vi "SV Read Spectra from Data Object.vi"(8 "error in (no error)":errorcluster, 10 "component":T1=32 items=["Magnitude^2"=37, "Magnitude"=32, "Phase"=33, "Real"=34, "Imaginary"=35, "Coherence"=36, "Unknown"=99], 11 "Data in":refnum<class "Data.lvclass">) -> (0 "error out":errorcluster, 1 "spectra info":T2[](array[typedef]) {"x-axis units" items=["Time (s)"=0, "Frequency-CB (Hz)"=1, "Frequency-CPB (Hz)"=1248, "Frequency-Arbitrary (Hz)"=2357, "Quefrency (s)"=2, "Revolutions (rev)"=3, "Order"=4, "Speed (RPM)"=11, "Speed (rad/s)"=21, "Index"=65535]; "weighting filter" items=["Linear", "A-weighting", "B-weighting", "C-weighting", "ITU-R 468-4", "Dolby", "CCITT", "C-message", "Wb", "Wc", "Wd", "We", "Wf", "Wh", "Wj", "Wk", "Wm", "AES17 20 kHz lowpass", "AES17 40 kHz lowpass", "AES17 20 kHz highpass", "AES17 40 kHz highpass"]; "dB reference [EU]" format="%.2f"; "engineering units" items=["custom..."=0, "V"=1, "A"=21, "C"=30, "pC"=31, "s"=32, "-"=29, "Pa"=2, "N"=20, "g"=3, "m/s^2"=4, "m/s"=5, "m"=6, "mm/s"=12, "mm"=13, "micron/s"=14, "micron"=15, "in/s^2"=7, "in/s"=8, "in"=9, "mil/s"=10, "mil"=11, "rad/s^2"=16, "rad/s"=17, "rad"=18, "deg/s^2"=26, "deg/s"=27, "deg"=28, "RPM"=22, "cycle/s^2"=23, "Hz"=24, "cycle"=25, "strain"=19]; "spectral info"."window" items=["None "=0, "Hanning"=1, "Hamming"=2, "Blackman-Harris"=3, "Exact Blackman"=4, "Blackman"=5, "Flat Top"=6, "4 Term B-Harris "=7, "7 Term B-Harris"=8, "Low Sidelobe"=9, "Force - Exponential"=10, "Gaussian"=62]}, 2 "spectra":cluster{"x0":dbl, "dx":dbl, "Y":dbl[]}[](array[cluster]), 3 "Data out":refnum<class "Data.lvclass">, 4 "global attributes":variant)   [LabVIEW 2017]
doc: "This VI always reads N Channel spectra from the data object."
uses:
  <vilib>/addons/_NISVFA/_Shared subVIs/Data Objects/Data/Data.lvclass
  <vilib>/addons/_NISVFA/_Shared subVIs/Controls/svc_Spectrum Info.ctl
  <vilib>/addons/_NISVFA/_Shared subVIs/Controls/svc_X-Axis Units.ctl
  <vilib>/addons/_NISVFA/_Shared subVIs/Controls/svc_Spectrum Type.ctl
  <vilib>/addons/_NISVFA/_Shared subVIs/Controls/svc_Engineering Units Text Ring.ctl
  <vilib>/addons/_NISVFA/_Shared subVIs/Controls/svc_Weighting Filter Text Ring.ctl
  <vilib>/addons/_NISVFA/_Shared subVIs/Controls/svc_Complimentary Spectrum Units.ctl
  <vilib>/addons/_NISVFA/_Shared subVIs/Controls/NI Spectrum Component.ctl
  <vilib>/addons/_NISVFA/_Shared subVIs/Controls/NI Channel Properties.ctl
  <vilib>/addons/_NISVFA/_Shared subVIs/Data Objects/Y (DBL)/Y (1 Ch).lvclass
  C:/Program Files (x86)/National Instruments/LabVIEW 2017/vi.lib/addons/_NISVFA/_Shared subVIs/Data Objects/Data/Data.lvclass
  <vilib>/addons/_NISVFA/_Shared subVIs/Data Objects/Data/Data.lvclass/Data.ctl
  <vilib>/addons/_NISVFA/_Shared subVIs/Data Objects/Y (DBL)/Y (N Ch).lvclass
  <vilib>/addons/_NISVFA/_Shared subVIs/Data Objects/Y (Complex) (DBL)/Y (Complex) (1 Ch).lvclass
  <vilib>/addons/_NISVFA/_Shared subVIs/Data Objects/Y (Complex) (DBL)/Y (Complex) (1 Ch).lvclass/Y (Complex) (1 Ch).ctl
  <vilib>/addons/_NISVFA/_Shared subVIs/Data Objects/Y (Complex) (DBL)/Y (Complex) (N Ch).lvclass
  <vilib>/addons/_NISVFA/_Shared subVIs/Data Objects/Y (Complex) (DBL)/Y (Complex) (N Ch).lvclass/Y (Complex) (N Ch).ctl
  <vilib>/addons/_NISVFA/_Shared subVIs/Common/sv_Get SV Property Name String.vi
  <vilib>/addons/_NISVFA/_Shared subVIs/Common/svc_Spectrum Units.vi
  <vilib>/addons/_NISVFA/_Shared subVIs/Spectrum Info/sfva_Set SV Info in Spectrum Info Description.vi
  <vilib>/addons/_NISVFA/_Shared subVIs/Common/svc_Get Weighting Enum and Labels.vi
  <vilib>/addons/_NISVFA/_Shared subVIs/Common/svc_Unit Label Lexical Class.vi
  <vilib>/addons/_NISVFA/_Shared subVIs/Common/svc_Engineering Units to Unit Label.vi
  <vilib>/addons/_NISVFA/_Shared subVIs/Common/svc_Format Value (DBL).vi
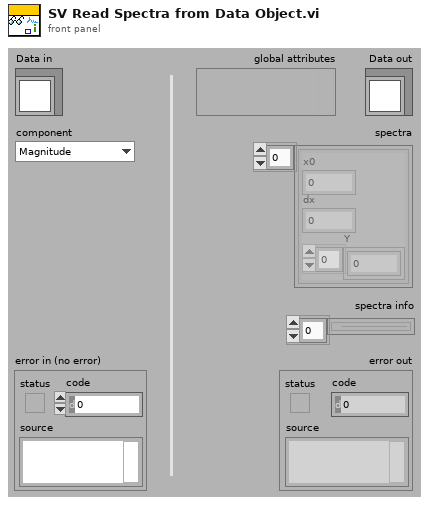
[diagram p1: front panel]
types:
  T1 = typedef "NI Spectrum Component.ctl" = u16
  T2 = typedef "svc_Spectrum Info.ctl" = cluster{"channel name":string, "description":string, "x-axis units":T3, "spectral info":cluster{"spectrum type":T4, "linear/dB":enum16{"linear", "dB"}, "window":u16, "window size":i32, "FFT size":i32}, "engineering units":T5, "custom label":string, "dB reference [EU]":dbl, "peak units":enum16{"rms", "peak", "peak-peak"}, "weighting filter":T6, "spectral density?":bool, "unit label":string, "spectrum skewed?":bool, "complimentary spectrum units":T7}
  T3 = typedef "svc_X-Axis Units.ctl" = u16
  T4 = typedef "svc_Spectrum Type.ctl" = enum16{"FFT Spectrum [complex]", "Amplitude [Magnitude]", "Power [Magnitude^2]", "Cross Spectrum [complex]", "Frequency Response [Complex]"}
  T5 = typedef "svc_Engineering Units Text Ring.ctl" = u16
  T6 = typedef "svc_Weighting Filter Text Ring.ctl" = u16
  T7 = typedef "svc_Complimentary Spectrum Units.ctl" = enum16{"none", "radians", "degrees", "cycles", "imaginary"}
  T8 = typedef "NI Channel Properties.ctl" = u16
  T9 = cluster{"Y":dbl[], "channel attributes":variant}[]
  T10 = cluster{"Y":cdb[], "channel attributes":variant}[]
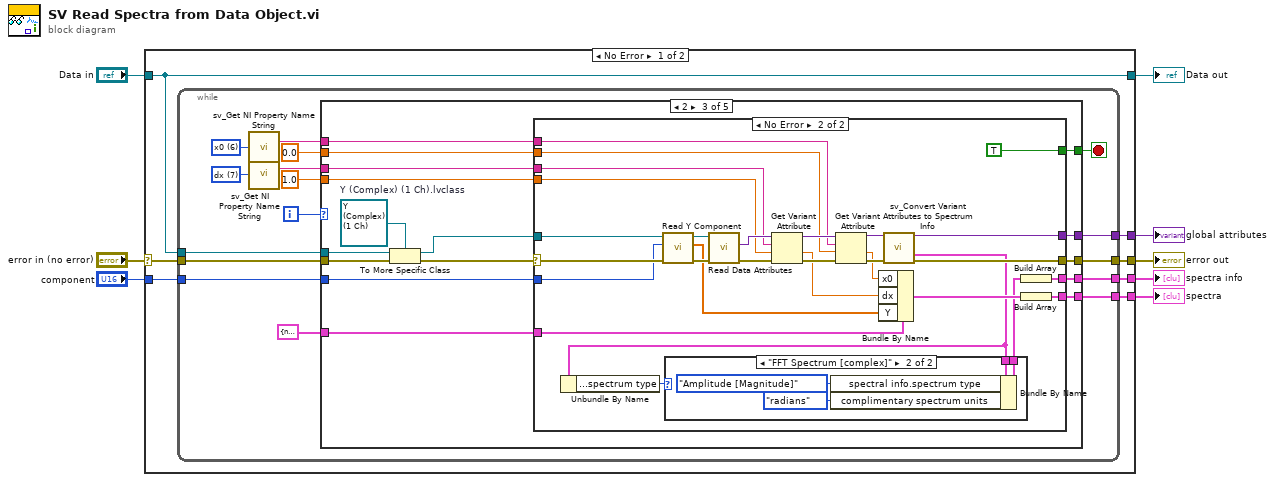
[diagram p0: block diagram]
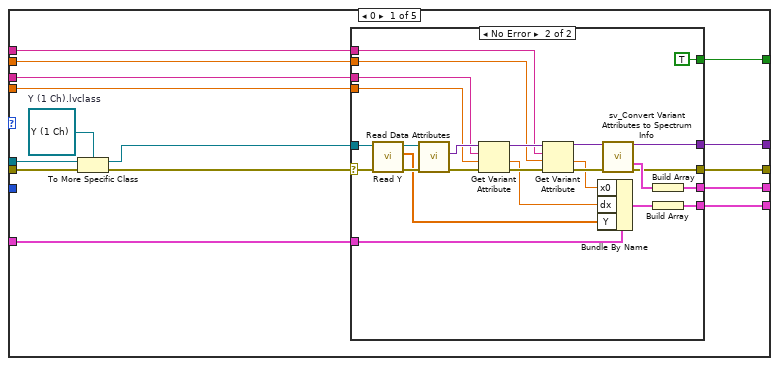
[diagram p2: hidden frame]
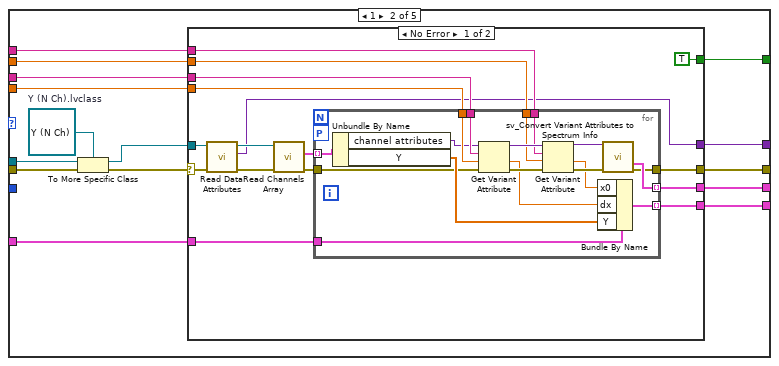
[diagram p4: hidden frame]
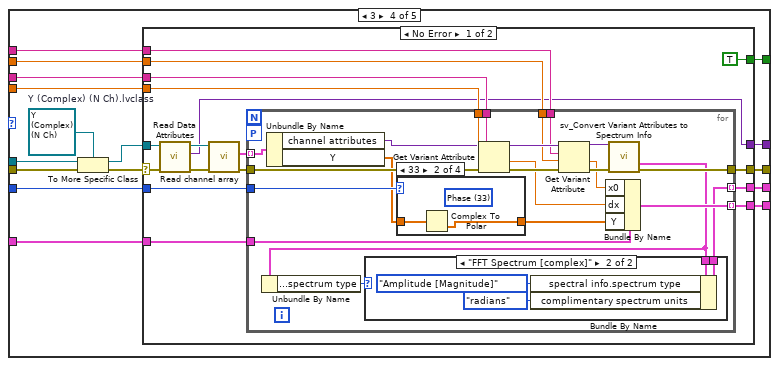
[diagram p8: hidden frame]
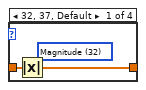
[diagram p10: hidden frame]
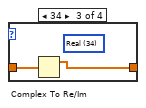
[diagram p11: hidden frame]
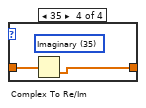
[diagram p12: hidden frame]
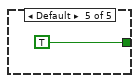
[diagram p14: hidden frame]
diagram:
  n1 = case shown="No Error" "error in (no error)" {
    selector: "error in (no error)" -> [w15 w243]
    tunnel: [w12 w243] -> w7
    tunnel: [w14 w244] -> w5
    tunnel: "Data in" -> [w14 w244]
    tunnel: [w13 _] -> w2
    tunnel: [w11 _] -> w4
    tunnel: [w10 _] -> w3
    tunnel: "component" -> [w9 _]
    frame No Error {
      n2 = while {
        tunnel: [w20] -> w12
        tunnel: w15 -> [w29]
        tunnel: w14 -> [w30]
        tunnel: [w21] -> w13
        tunnel: [w19] -> w11
        tunnel: [w18] -> w10
        tunnel: w9 -> [w16]
        i -> [w31]
        stop <- w17 stop-if-true
        w28 = T8 7 items=["Channel name", "Channel description", "Y-axis label", "Y-axis unit string", "X-axis label", "X-axis unit string", "x0", "dx", "Number of samples", "X channel", "Filter settled", "dB reference", "Window", "Window parameter", "Window size", "FFT size", "Peak units", "Spectrum type", "Magnitude scale", "Spectral density"] ("property")
        w27 = T8 6 items=["Channel name", "Channel description", "Y-axis label", "Y-axis unit string", "X-axis label", "X-axis unit string", "x0", "dx", "Number of samples", "X channel", "Filter settled", "dB reference", "Window", "Window parameter", "Window size", "FFT size", "Peak units", "Spectrum type", "Magnitude scale", "Spectral density"] ("property")
        n3 = call <vilib>:"sv_Get NI Property Name String.vi"("property"=w27) -> ("TDMS property name"=w26:string)  [unwired: 13 in, 1 out]
        n4 = call <vilib>:"sv_Get NI Property Name String.vi"("property"=w28) -> ("TDMS property name"=w24:string)  [unwired: 13 in, 1 out]
        n5 = case shown="2" w31 {
          tunnel: w30 -> [w45 w86 w137 w187 _]
          tunnel: w29 -> [w44 w85 w136 w186 _]
          tunnel: w26 -> [w43 w82 w135 w183 _]
          tunnel: 0.0 -> [w42 w81 w134 w182 _]
          tunnel: w24 -> [w41 w80 w133 w181 _]
          tunnel: 1.0 -> [w40 w79 w132 w180 _]
          tunnel: cluster{"x0":dbl, "dx":dbl, "Y":dbl[]} {"x0"=nan, "dx"=nan, "Y"=[nan]} ("power spectrum [dB EU]") -> [w39 w78 w131 w179 _]
          tunnel: [w36 w74 w128 w175 _] -> w21
          tunnel: [w35 w75 w127 w176 _] -> w20
          tunnel: [w34 w76 w126 w177 _] -> w19
          tunnel: [w33 w77 w125 w178 _] -> w18
          tunnel: [w32 w73 w124 w174 TRUE] -> w17
          tunnel: w16 -> [_ _ w123 w173 _]
          frame 0 {
            w46 = refnum<class "Y (1 Ch).lvclass"> refnum  # Y (1 Ch).lvclass
            n6 = To More Specific Class(target class=w46, reference=w45, error in=w44) -> (specific class reference=w37:refnum<class "Y (1 Ch).lvclass">, error out=w38:errorcluster)
            n7 = case shown="No Error" w38 {
              selector: w38 -> [w47 w52]
              tunnel: w37 -> [_ w61]
              tunnel: [_ w53] -> w34
              tunnel: w43 -> [_ w60]
              tunnel: w41 -> [_ w58]
              tunnel: w40 -> [_ w57]
              tunnel: w42 -> [_ w59]
              tunnel: w39 -> [_ w56]
              tunnel: [_ w55] -> w33
              tunnel: [w47 w51] -> w35
              tunnel: [_ w50] -> w36
              tunnel: [_ TRUE] -> w32
              frame Error {
              }
              frame No Error {
                n8 = call <vilib>:"Read Y.vi"("error in (no error)"=w52, "Y (1Ch) in"=w61) -> ("error out"=w67:errorcluster, "Y"=w62:dbl[], "Y (1Ch) out"=w72:refnum<class "Y (1 Ch).lvclass">)  [unwired: 7 in]
                n9 = call <vilib>:"Read Data Attributes.vi"("error in (no error)"=w67, "Data in"=w72) -> ("error out"=w68:errorcluster, "data attributes"=w69:variant)  [unwired: 7 in, 1 out]
                n10 = Get Variant Attribute(Variant=w69, name=w58, default value (empty Variant)=w57, error in=w68) -> (duplicate Variant=w70:variant, value=w63:dbl, error out=w71:errorcluster)  [unwired: 1 out]
                n11 = Get Variant Attribute(Variant=w70, name=w60, default value (empty Variant)=w59, error in=w71) -> (duplicate Variant=w66:variant, value=w64:dbl, error out=w65:errorcluster)  [unwired: 1 out]
                n12 = Bundle By Name(cluster=w56, "x0"=w64, "dx"=w63, "Y"=w62) -> (w49:cluster{"x0":dbl, "dx":dbl, "Y":dbl[]})
                n13 = call <vilib>:"sv_Convert Variant Attributes to Spectrum Info.vi"("variant attributes"=w66, "error in"=w65) -> ("variant attributes"=w50:variant, "spectrum info"=w54:T2, "error out"=w51:errorcluster)  [unwired: 11 in]
                n14 = Build Array(w54) -> (w53:T2[])
                n15 = Build Array(w49) -> (w55:cluster{"x0":dbl, "dx":dbl, "Y":dbl[]}[])
              }
            }
          }
          frame 1 {
            w87 = refnum<class "Y (N Ch).lvclass"> refnum  # Y (N Ch).lvclass
            n16 = To More Specific Class(target class=w87, reference=w86, error in=w85) -> (specific class reference=w83:refnum<class "Y (N Ch).lvclass">, error out=w84:errorcluster)
            n17 = case shown="No Error" w84 {
              selector: w84 -> [w92 w122]
              tunnel: w83 -> [w93 _]
              tunnel: [w102 _] -> w76
              tunnel: w82 -> [w101 _]
              tunnel: w80 -> [w100 _]
              tunnel: w79 -> [w99 _]
              tunnel: w81 -> [w98 _]
              tunnel: w78 -> [w97 _]
              tunnel: [w96 _] -> w77
              tunnel: [w95 w122] -> w75
              tunnel: [w89 _] -> w74
              tunnel: [TRUE _] -> w73
              frame No Error {
                n18 = call <vilib>:"Read Data Attributes.vi"("error in (no error)"=w92, "Data in"=w93) -> ("error out"=w90:errorcluster, "data attributes"=w89:variant, "Data out"=w91:refnum<class "Y (N Ch).lvclass">)  [unwired: 7 in]
                n19 = call <vilib>:"Read Channels Array.vi"("error in (no error)"=w90, "Y (N Ch) in"=w91) -> ("error out"=w103:errorcluster, "channel array"=w94:T9)  [unwired: 7 in, 1 out]
                n20 = for {
                  tunnel: w101 -> [w119]
                  tunnel: w103 -> [w104]
                  tunnel: [w116] -> w102 mode=indexing
                  tunnel: w100 -> [w115]
                  tunnel: w99 -> [w114]
                  tunnel: w98 -> [w113]
                  tunnel: w97 -> [w112]
                  tunnel: [w109] -> w96 mode=indexing
                  tunnel: [w108] -> w95
                  tunnel: w94 -> [w107] mode=indexing
                  workers-P: _ -> [_]
                  n21 = Unbundle By Name(w107) -> ("channel attributes"=w106:variant, "Y"=w105:dbl[])
                  n22 = Get Variant Attribute(Variant=w106, name=w115, default value (empty Variant)=w114, error in=w104) -> (duplicate Variant=w120:variant, value=w110:dbl, error out=w121:errorcluster)  [unwired: 1 out]
                  n23 = Get Variant Attribute(Variant=w120, name=w119, default value (empty Variant)=w113, error in=w121) -> (duplicate Variant=w118:variant, value=w111:dbl, error out=w117:errorcluster)  [unwired: 1 out]
                  n24 = Bundle By Name(cluster=w112, "x0"=w111, "dx"=w110, "Y"=w105) -> (w109:cluster{"x0":dbl, "dx":dbl, "Y":dbl[]})
                  n25 = call <vilib>:"sv_Convert Variant Attributes to Spectrum Info.vi"("variant attributes"=w118, "error in"=w117) -> ("spectrum info"=w116:T2, "error out"=w108:errorcluster)  [unwired: 11 in, 1 out]
                }
              }
              frame Error {
              }
            }
          }
          frame 2 {
            w138 = refnum<class "Y (Complex) (1 Ch).lvclass"> refnum  # Y (Complex) (1 Ch).lvclass
            n26 = To More Specific Class(target class=w138, reference=w137, error in=w136) -> (specific class reference=w129:refnum<class "Y (Complex) (1 Ch).lvclass">, error out=w130:errorcluster)
            n27 = case shown="No Error" w130 {
              selector: w130 -> [w139 w148]
              tunnel: w129 -> [_ w156]
              tunnel: [_ w149] -> w126
              tunnel: w135 -> [_ w155]
              tunnel: w133 -> [_ w153]
              tunnel: w132 -> [_ w152]
              tunnel: w134 -> [_ w154]
              tunnel: w131 -> [_ w151]
              tunnel: [_ w150] -> w125
              tunnel: [w139 w147] -> w127
              tunnel: [_ w146] -> w128
              tunnel: [_ TRUE] -> w124
              tunnel: w123 -> [_ w142]
              frame Error {
              }
              frame No Error {
                n28 = call <vilib>:"Read Y Component.vi"("error in (no error)"=w148, "component"=w142, "Y (Complex) (1Ch) in"=w156) -> ("error out"=w162:errorcluster, "Y"=w157:dbl[], "Y (Complex) (1Ch) out"=w167:refnum<class "Y (Complex) (1 Ch).lvclass">)  [unwired: 6 in]
                n29 = call <vilib>:"Read Data Attributes.vi"("error in (no error)"=w162, "Data in"=w167) -> ("error out"=w163:errorcluster, "data attributes"=w164:variant)  [unwired: 7 in, 1 out]
                n30 = Get Variant Attribute(Variant=w164, name=w153, default value (empty Variant)=w152, error in=w163) -> (duplicate Variant=w165:variant, value=w158:dbl, error out=w166:errorcluster)  [unwired: 1 out]
                n31 = Get Variant Attribute(Variant=w165, name=w155, default value (empty Variant)=w154, error in=w166) -> (duplicate Variant=w161:variant, value=w159:dbl, error out=w160:errorcluster)  [unwired: 1 out]
                n32 = Bundle By Name(cluster=w151, "x0"=w159, "dx"=w158, "Y"=w157) -> (w145:cluster{"x0":dbl, "dx":dbl, "Y":dbl[]})
                n33 = call <vilib>:"sv_Convert Variant Attributes to Spectrum Info.vi"("variant attributes"=w161, "error in"=w160) -> ("variant attributes"=w146:variant, "spectrum info"=w141:T2, "error out"=w147:errorcluster)  [unwired: 11 in]
                n34 = Unbundle By Name(w141) -> ("spectral info.spectrum type"=w140:T4)
                n35 = case shown="\"FFT Spectrum [complex]\"" w140 {
                  tunnel: [w168 w172] -> w143
                  tunnel: w141 -> [w168 w170]
                  frame Default {
                  }
                  frame "FFT Spectrum [complex]" {
                    n36 = Bundle By Name(cluster=w170, "spectral info.spectrum type"=svc_Spectrum_Type."Amplitude [Magnitude]", "complimentary spectrum units"=svc_Complimentary_Spectrum_Units."radians") -> (w172:T2)
                  }
                }
                n37 = Build Array(w143) -> (w149:T2[])
                n38 = Build Array(w145) -> (w150:cluster{"x0":dbl, "dx":dbl, "Y":dbl[]}[])
              }
            }
          }
          frame 3 {
            w188 = refnum<class "Y (Complex) (N Ch).lvclass"> refnum  # Y (Complex) (N Ch).lvclass
            n39 = To More Specific Class(target class=w188, reference=w187, error in=w186) -> (specific class reference=w184:refnum<class "Y (Complex) (N Ch).lvclass">, error out=w185:errorcluster)
            n40 = case shown="No Error" w185 {
              selector: w185 -> [w194 w241]
              tunnel: w184 -> [w195 _]
              tunnel: [w204 _] -> w177
              tunnel: w183 -> [w203 _]
              tunnel: w181 -> [w202 _]
              tunnel: w180 -> [w201 _]
              tunnel: w182 -> [w200 _]
              tunnel: w179 -> [w199 _]
              tunnel: [w198 _] -> w178
              tunnel: [w197 w241] -> w176
              tunnel: [w191 _] -> w175
              tunnel: [TRUE _] -> w174
              tunnel: w173 -> [w189 _]
              frame No Error {
                n41 = call <vilib>:"Read Data Attributes.vi"("error in (no error)"=w194, "Data in"=w195) -> ("error out"=w192:errorcluster, "data attributes"=w191:variant, "Data out"=w193:refnum<class "Y (Complex) (N Ch).lvclass">)  [unwired: 7 in]
                n42 = call <vilib>:"Read channel array.vi"("error in (no error)"=w192, "Y (Complex) (N Ch) in"=w193) -> ("error out"=w205:errorcluster, "channel array"=w196:T10)  [unwired: 7 in, 1 out]
                n43 = for {
                  tunnel: w203 -> [w225]
                  tunnel: w205 -> [w212]
                  tunnel: [w207] -> w204 mode=indexing
                  tunnel: w202 -> [w222]
                  tunnel: w201 -> [w221]
                  tunnel: w200 -> [w220]
                  tunnel: w199 -> [w219]
                  tunnel: [w216] -> w198 mode=indexing
                  tunnel: [w215] -> w197
                  tunnel: w196 -> [w214] mode=indexing
                  workers-P: _ -> [_]
                  tunnel: w189 -> [w211]
                  n44 = Unbundle By Name(w214) -> ("channel attributes"=w213:variant, "Y"=w209:cdb[])
                  n45 = case shown="33" w211 {
                    tunnel: w209 -> [w234 w236 w238 w240]
                    tunnel: [w233 w235 w237 w239] -> w210
                    frame 32, 37, Default {
                      (unwired) T1 32 items=["Magnitude"=32, "Phase"=33, "Real"=34, "Imaginary"=35, "Coherence"=36, "Unknown"=99] ("component")
                      n46 = Absolute Value(x=w234) -> (abs(x)=w233:dbl[])
                    }
                    frame 33 {
                      (unwired) T1 33 items=["Magnitude"=32, "Phase"=33, "Real"=34, "Imaginary"=35, "Coherence"=36, "Unknown"=99] ("component")
                      n47 = Complex To Polar(r * e^(i*theta)=w236) -> (theta=w235:dbl[])  [unwired: 1 out]
                    }
                    frame 34 {
                      (unwired) T1 34 items=["Magnitude"=32, "Phase"=33, "Real"=34, "Imaginary"=35, "Coherence"=36, "Unknown"=99] ("component")
                      n48 = Complex To Re/Im(x + iy=w238) -> (x=w237:dbl[])  [unwired: 1 out]
                    }
                    frame 35 {
                      (unwired) T1 35 items=["Magnitude"=32, "Phase"=33, "Real"=34, "Imaginary"=35, "Coherence"=36, "Unknown"=99] ("component")
                      n49 = Complex To Re/Im(x + iy=w240) -> (y=w239:dbl[])  [unwired: 1 out]
                    }
                  }
                  n50 = Get Variant Attribute(Variant=w213, name=w222, default value (empty Variant)=w221, error in=w212) -> (duplicate Variant=w226:variant, value=w217:dbl, error out=w227:errorcluster)  [unwired: 1 out]
                  n51 = Get Variant Attribute(Variant=w226, name=w225, default value (empty Variant)=w220, error in=w227) -> (duplicate Variant=w224:variant, value=w218:dbl, error out=w223:errorcluster)  [unwired: 1 out]
                  n52 = Bundle By Name(cluster=w219, "x0"=w218, "dx"=w217, "Y"=w210) -> (w216:cluster{"x0":dbl, "dx":dbl, "Y":dbl[]})
                  n53 = call <vilib>:"sv_Convert Variant Attributes to Spectrum Info.vi"("variant attributes"=w224, "error in"=w223) -> ("spectrum info"=w208:T2, "error out"=w215:errorcluster)  [unwired: 11 in, 1 out]
                  n54 = Unbundle By Name(w208) -> ("spectral info.spectrum type"=w206:T4)
                  n55 = case shown="\"FFT Spectrum [complex]\"" w206 {
                    tunnel: [w228 w232] -> w207
                    tunnel: w208 -> [w228 w230]
                    frame Default {
                    }
                    frame "FFT Spectrum [complex]" {
                      n56 = Bundle By Name(cluster=w230, "spectral info.spectrum type"=svc_Spectrum_Type."Amplitude [Magnitude]", "complimentary spectrum units"=svc_Complimentary_Spectrum_Units."radians") -> (w232:T2)
                    }
                  }
                }
              }
              frame Error {
              }
            }
          }
          frame Default {
          }
        }
      }
    }
    frame Error {
    }
  }
  "error out" <- w7
  "Data out" <- w5
  "spectra info" <- w4
  "spectra" <- w3
  "global attributes" <- w2
